vi "calculo covariância.vi"(10 "cluster":cluster{"f1":dbl, "f2":dbl}, 11 "Array":cluster{"f1":dbl, "f2":dbl}[](array[cluster])) -> (3 "element":dbl)   [LabVIEW 2014]
uses:
  <vilib>/Analysis/Matrix/Datatypes/RealMatrix.ctl
  <vilib>/Analysis/Matrix/Numeric/Conversions/Array To Matrix - RA.vi
  <vilib>/Analysis/baseanly.llb/Real Inverse Matrix.vi
  <vilib>/Analysis/Matrix/Numeric/Multiply/Multiply - RM,RM.vi
  <vilib>/Analysis/NI_AALBase.lvlib
  <vilib>/gmath/NI_Gmath.lvlib
  <vilib>/Analysis/Matrix/NI_Matrix.lvlib
panel:
  out "Real Matrix (Column Vector)":T1
  out "covariance matrix V":T1
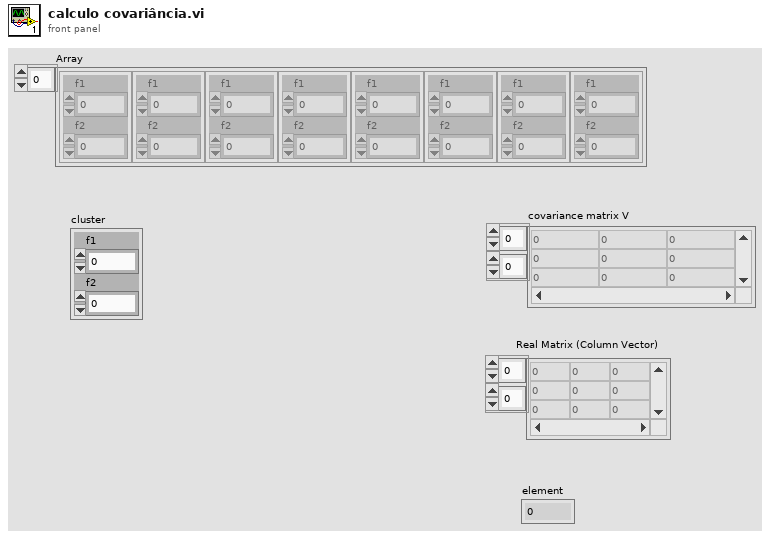
[diagram p1: front panel]
types:
  T1 = typedef "NI_Matrix.lvlib/RealMatrix.ctl" = dbl[][]
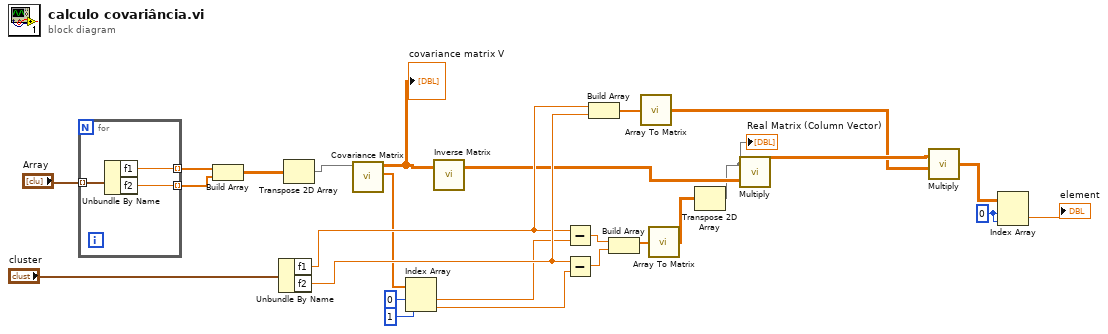
[diagram p0: block diagram]
diagram:
  w4 = 0 ("index (row)")
  n1 = for {
    tunnel: "Array" -> [w29] mode=indexing
    tunnel: [w28] -> w8 mode=indexing
    tunnel: [w27] -> w9 mode=indexing
    n2 = Unbundle By Name(w29) -> ("f1"=w28:dbl, "f2"=w27:dbl)
  }
  n3 = Build Array(w8, w9) -> (w12:dbl[][])
  n4 = Unbundle By Name("cluster") -> ("f1"=w25:dbl, "f2"=w26:dbl)
  n5 = Transpose 2D Array(2D array=w12) -> (transposed array=w13:dbl[][])
  n6 = call <vilib>:"Covariance Matrix.vi"("X"=w13) -> ("mean vector"=w14:dbl[], "covariance matrix V"=w19:T1)  [unwired: 9 in]
  "covariance matrix V" <- w19
  n7 = Index Array(array=w14, index #1=0 ("index"), index #2=1 ("index")) -> (element #1=w17:dbl, element #2=w18:dbl)
  n8 = call-poly <vilib>:"Inverse Matrix.vi"("Input Matrix"=w19) -> ("Inverse Matrix"=w21:T1)  [unwired: 1 in, 1 out]
  n9 = Subtract(x=w25, y=w17) -> (x-y=w10:dbl)
  n10 = Subtract(x=w26, y=w18) -> (x-y=w11:dbl)
  n11 = Build Array(w25, w26) -> (w24:dbl[])
  n12 = Build Array(w10, w11) -> (w22:dbl[])
  n13 = call-poly <vilib>:"Array To Matrix.vi"("Real 1D Array"=w24) -> ("Real Matrix (Column Vector)"=w1:T1)
  n14 = call-poly <vilib>:"Array To Matrix.vi"("Real 1D Array"=w22) -> ("Real Matrix (Column Vector)"=w23:T1)
  n15 = Transpose 2D Array(2D array=w23) -> (transposed array=w6:T1)
  "Real Matrix (Column Vector)" <- w6
  n16 = call-poly <vilib>:"Multiply.vi"("Real Matrix B"=w21, "Real Matrix A"=w6) -> ("A * B"=w2:T1)
  n17 = call-poly <vilib>:"Multiply.vi"("Real Matrix B"=w1, "Real Matrix A"=w2) -> ("A * B"=w5:T1)
  n18 = Index Array(array=w5, index (row)=w4, index (col)=w4) -> (element=→"element":dbl)
